vi "OpenCV UnsharpMask.vi"(8 "error in (no error)":errorcluster, 9 "Unsharp Mask Params":T1={"Amount"=6.0, "Radius"=33.0, "Threshold"=30.0}, 10 "Image Dst":T2, 11 "Image Src":T2) -> (0 "error out":errorcluster, 1 "time, ms":u32, 3 "Image Dst Out":T2)   [LabVIEW 2023]
uses:
  <vilib>/vision/Image Controls.llb/IMAQ Image.ctl
  SubVIs/Unsharp Mask Params TypeDef.ctl
  WrapperDLL/x64/Release/Wrapper.dll
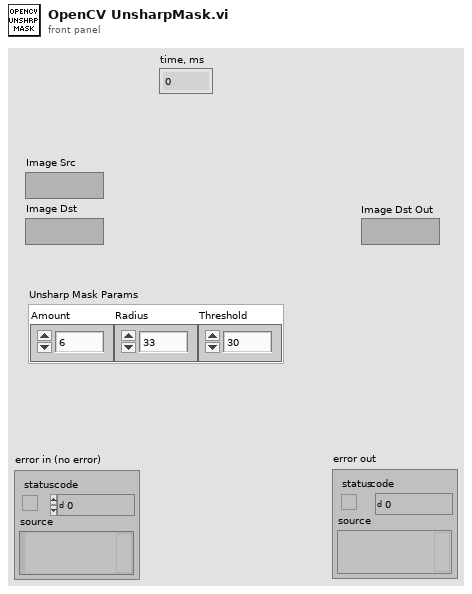
[diagram p1: front panel]
types:
  T1 = typedef "Unsharp Mask Params TypeDef.ctl" = cluster{"Amount":sgl, "Radius":sgl, "Threshold":sgl}
  T2 = typedef "IMAQ Image.ctl" = refnum<image>
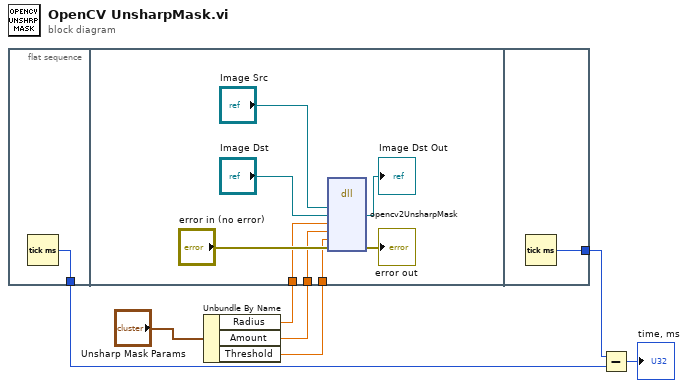
[diagram p0: block diagram]
diagram:
  n1 = flat-sequence {
    tunnel: [w8] -> w6
    tunnel: w2 -> [w11]
    tunnel: w1 -> [w10]
    tunnel: w3 -> [w9]
    tunnel: [w17] -> w7
    frame #0 {
      n2 = Tick Count (ms)() -> (millisecond timer value=w8:u32)
    }
    frame #1 {
      n3 = dll-call lib="C:/Users/Andrey/Desktop/xe2/WrapperDLL/x64/Release/Wrapper.dll" fn="opencv2UnsharpMask"("src"="Image Src", "dst"="Image Dst", "Radius"=w11, "Amount"=w10, "Threshold"=w9, "error"="error in (no error)") -> ("dst"=→"Image Dst Out":T2, "error"=→"error out":errorcluster)  [unwired: 8 in, 2 out]
    }
    frame #2 {
      n4 = Tick Count (ms)() -> (millisecond timer value=w17:u32)
    }
  }
  n5 = Unbundle By Name("Unsharp Mask Params") -> ("Radius"=w2:sgl, "Amount"=w1:sgl, "Threshold"=w3:sgl)
  n6 = Subtract(x=w7, y=w6) -> (x-y=→"time, ms":u32)
